vi "Configure Channel.vi"(8 "error in (no error)":errorcluster, 10 "DAQmx Task In":refnum<k21>, 11 "CurrentOutChannel in":refnum<class "CurrentOutChannel.lvclass">) -> (0 "error out":errorcluster, 2 "DAQmx Task":refnum<k21>)   [LabVIEW 2020, in "VolatusDAQConfig.lvlib" / "CurrentOutChannel.lvclass"]
uses:
  CurrentOutChannel.lvclass
  CurrentOutChannel.lvclass/CurrentOutChannel.ctl
  VolatusConfig/VolatusConfigElement/VolatusConfigElement.lvclass
  VolatusConfig/Channel/Channel.lvclass
  C:/dev/lv20CE/relink/lv-volatus/VolatusDAQConfig/DAQmxChannel/DAQmxChannel.lvclass
  C:/dev/lv20CE/relink/lv-volatus/VolatusConfig/Channel/Channel.lvclass
  C:/dev/lv20CE/relink/lv-volatus/VolatusConfig/VolatusConfigElement/VolatusConfigElement.lvclass
  C:/dev/lv20CE/relink/lv-volatus/VolatusDAQConfig/CurrentOutChannel/CurrentOutChannel.lvclass
  <vilib>/DAQmx/create/channels.llb/DAQmx Create Channel (AO-Current-Basic).vi
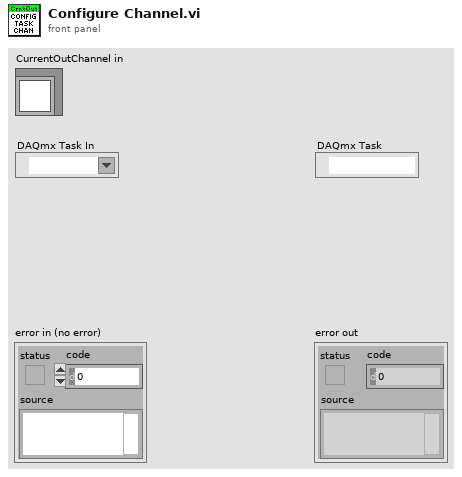
[diagram p1: front panel]
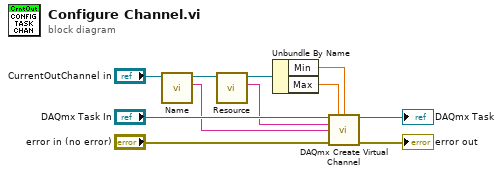
[diagram p0: block diagram]
diagram:
  n1 = call "Name.vi"("VolatusConfigElement in"="CurrentOutChannel in") -> ("Name"=w5:string, "VolatusConfigElement out"=w6:refnum<class "CurrentOutChannel.lvclass">)  [unwired: 8 in, 1 out]
  n2 = call "Resource.vi"("Channel in"=w6) -> ("Resource"=w4:string, "Channel out"=w3:refnum<class "CurrentOutChannel.lvclass">)  [unwired: 8 in, 1 out]
  n3 = Unbundle By Name(w3) -> ("Min"=w1:dbl, "Max"=w2:dbl)
  n4 = call-poly <vilib>:"DAQmx Create Virtual Channel.vi"("task in"="DAQmx Task In", "maximum value"=w2, "minimum value"=w1, "physical channels"=w4, "name to assign"=w5, "error in"="error in (no error)") -> ("task out"=→"DAQmx Task":refnum<k21>, "error out"=→"error out":errorcluster)  [unwired: 8 in]
